vi "Sampling.vi"(8 "No of Avg":i32, 11 "Unsampled":dbl[](array[numeric])) -> (0 "x+y":dbl[](array[numeric]), 3 "mean":dbl[](array[numeric]) format="%0.2f")   [LabVIEW 2017]
uses:
  <vilib>/Analysis/baseanly.llb/Mean (DBL).vi
  <vilib>/Analysis/NI_AALBase.lvlib
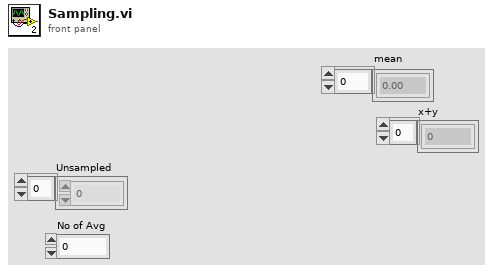
[diagram p1: front panel]
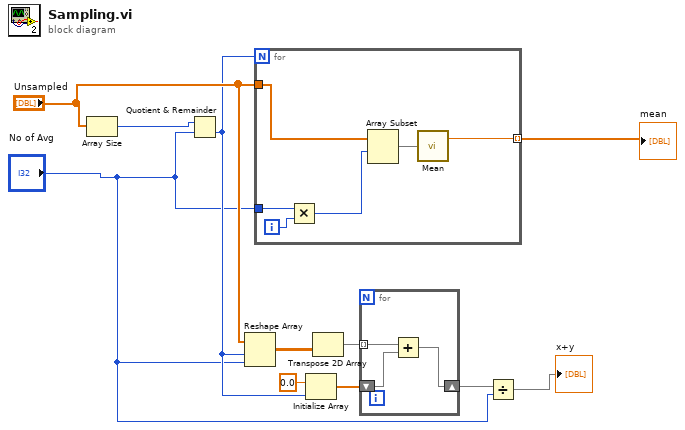
[diagram p0: block diagram]
diagram:
  n1 = Array Size(array="Unsampled") -> (size(s)=w11:i32)
  n2 = Quotient & Remainder(x=w11, y="No of Avg") -> (floor(x/y)=w6:i32)  [unwired: 1 out]
  n3 = Reshape Array("Unsampled", w6, "No of Avg") -> (w8:dbl[][])
  n4 = for {
    N: w6 -> [_]
    tunnel: "No of Avg" -> [w16]
    tunnel: "Unsampled" -> [w14]
    tunnel: [w12] -> w10 mode=indexing
    i -> [w17]
    n5 = Multiply(x=w16, y=w17) -> (x*y=w15:i32)
    n6 = Array Subset(array=w14, index=w15) -> (w13:dbl[])  [unwired: 1 in]
    n7 = call-poly <vilib>:"Mean.vi"("X"=w13) -> ("mean"=w12:dbl)  [unwired: 1 out]
  }
  "mean" <- w10
  n8 = Initialize Array(0.0 ("element"), w6) -> (w4:dbl[])
  n9 = Transpose 2D Array(2D array=w8) -> (transposed array=w9:dbl[][])
  n10 = for {
    tunnel: w9 -> [w20] mode=indexing
    shift-right: [w18] -> w3
    shift-left: w4 -> [w19]
    n11 = Add(x=w20, y=w19) -> (x+y=w18:dbl[])
  }
  n12 = Divide(x=w3, y="No of Avg") -> (x/y=→"x+y":dbl[])
